vi "Compare to Last.vi"(8 "error in (no error)":errorcluster, 10 "Joystick State Before Previous":T1, 11 "Joystick in":refnum<class "Joystick.lvclass">) -> (0 "error out":errorcluster, 2 "Joystick State With Previous":T1, 3 "Joystick out":refnum<class "Joystick.lvclass">)   [LabVIEW 2014, in "Joystick.lvlib" / "Joystick.lvclass"]
uses:
  Joystick.lvclass
  Joystick State.ctl
  Button State.ctl
  Axis State.ctl
  Joystick.lvclass/Joystick.ctl
panel:
  out "This Pressed":bool
  out "Last Pressed":bool
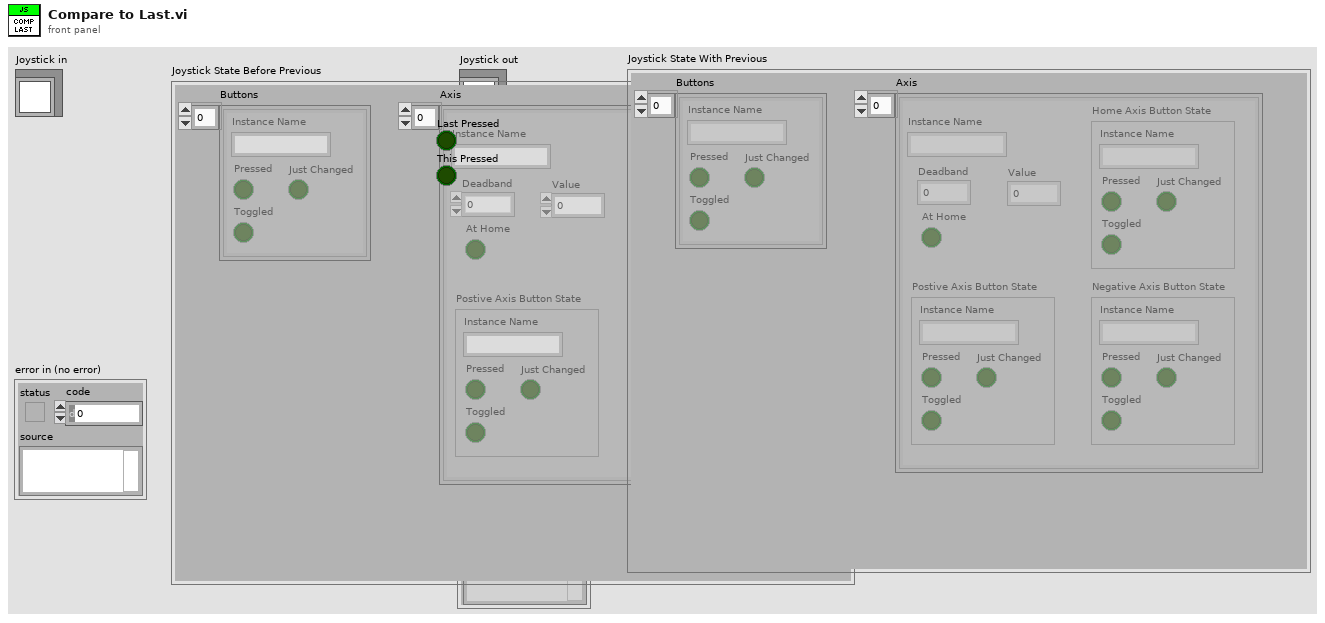
[diagram p1: front panel]
types:
  T1 = typedef "Joystick.lvlib/Joystick.lvclass/Joystick State.ctl" = cluster{"Buttons":T2[], "Axis":T3[]}
  T2 = typedef "Joystick.lvlib/Joystick.lvclass/Button State.ctl" = cluster{"Pressed":bool, "Instance Name":string, "Toggled":bool, "Just Changed":bool}
  T3 = typedef "Joystick.lvlib/Joystick.lvclass/Axis State.ctl" = cluster{"Instance Name":string, "Deadband":dbl, "Value":dbl, "At Home":bool, "Postive Axis Button State":T2, "Negative Axis Button State":T2, "Home Axis Button State":T2}
  T4 = typedef "Joystick.lvlib/Joystick.lvclass/Axis State.ctl" = cluster{"Instance Name":string, "Deadband":dbl, "Value":dbl, "At Home":bool}
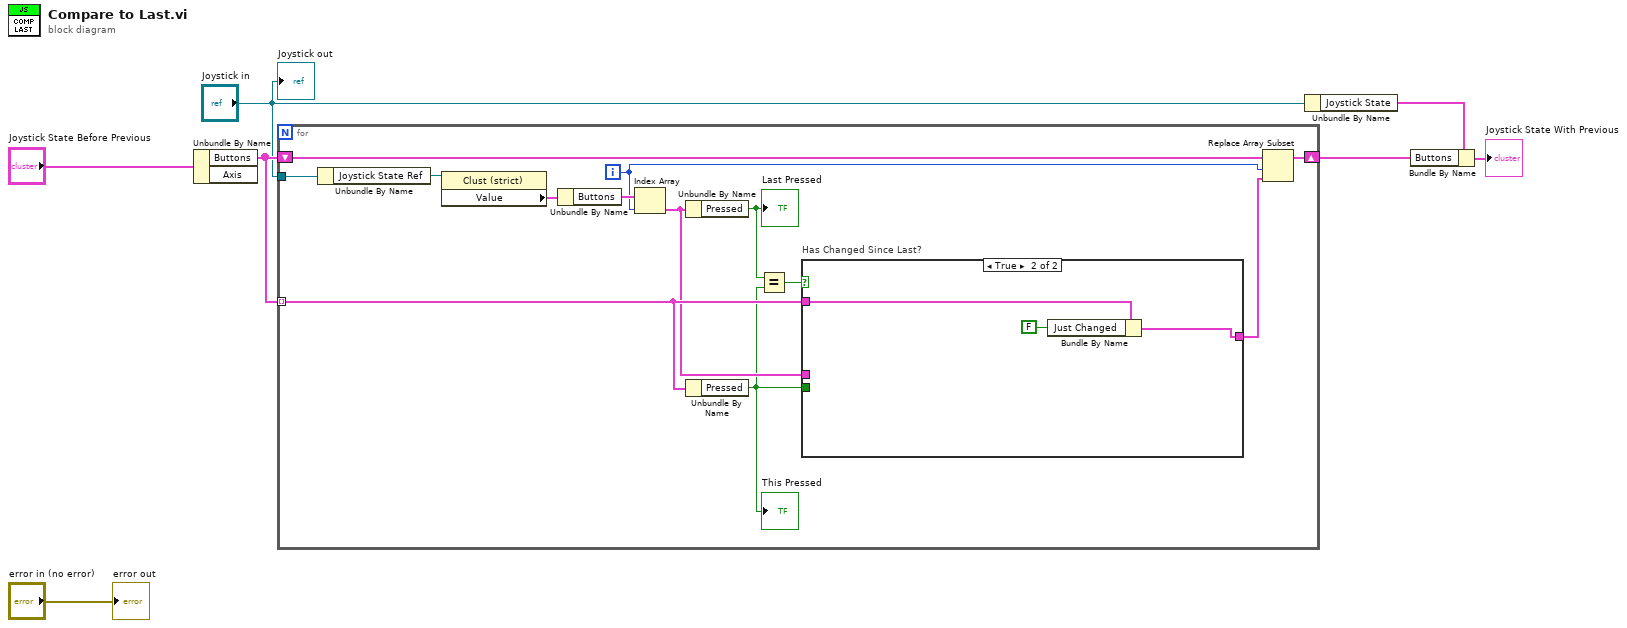
[diagram p0: block diagram]
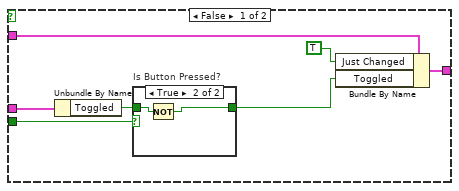
[diagram p2: hidden frame]
diagram:
  n1 = Unbundle By Name("Joystick State Before Previous") -> ("Buttons"=w5:T2[])  [unwired: 1 out]
  n2 = for {
    tunnel: "Joystick in" -> [w20]
    shift-right: [w15] -> w4
    shift-left: w5 -> [w13]
    tunnel: w5 -> [w14] mode=indexing
    i -> [w16]
    n3 = Unbundle By Name(w20) -> ("Joystick State Ref"=w19:refnum<vi>)
    n4 = property class="Clust (strict)"(reference=w19) -> ("Value"=w18:cluster{"Buttons":T2[], "Axis":T4[]})  [unwired: 1 in, 2 out]
    n5 = Unbundle By Name(w18) -> ("Buttons"=w17:T2[])
    n6 = Index Array(array=w17, index=w16) -> (element=w12:T2)
    n7 = Unbundle By Name(w12) -> ("Pressed"=w10:bool)
    "Last Pressed" <- w10
    n8 = Unbundle By Name(w14) -> ("Pressed"=w9:bool)
    "This Pressed" <- w9
    n9 = Equal?(x=w10, y=w9) -> (x = y?=w8:bool)
    n10 = case "Has Changed Since Last?" shown="True" w8 {
      tunnel: w14 -> [w24 w33]
      tunnel: [w26 w32] -> w11
      tunnel: w9 -> [w25 _]
      tunnel: w12 -> [w22 _]
      frame False {
        n11 = Unbundle By Name(w22) -> ("Toggled"=w23:bool)
        n12 = case "Is Button Pressed?" shown="True" w25 {
          tunnel: w23 -> [w28 w30]
          tunnel: [w28 w29] -> w21
          frame False {
          }
          frame True {
            n13 = Not(x=w30) -> (.not. x?=w29:bool)
          }
        }
        n14 = Bundle By Name(cluster=w24, "Just Changed"=TRUE, "Toggled"=w21) -> (w26:T2)
      }
      frame True {
        n15 = Bundle By Name(cluster=w33, "Just Changed"=FALSE) -> (w32:T2)
      }
    }
    n16 = Replace Array Subset(array=w13, new element=w11, index=w16) -> (w15:T2[])
  }
  n17 = Unbundle By Name("Joystick in") -> ("Joystick State"=w1:T1)
  n18 = Bundle By Name(cluster=w1, "Buttons"=w4) -> (→"Joystick State With Previous":T1)
  "error out" <- "error in (no error)"
  "Joystick out" <- "Joystick in"
